vi "TLEparsing.vi"(1 "String 2":string, 2 "String":string) -> (0 "parametres_TLE":cdb[][](array[numeric]))   [LabVIEW 2015]
uses:
  <vilib>/imath/engines/lvmath/Plug In/_Char/NIMS_CH_character datatype.ctl
  <vilib>/imath/engines/lvmath2/RunTimeEngine/Managers/WorkSpace/UID Generator.vi
  <vilib>/imath/engines/lvmath/Plug In/_Char/NIMS_CH_String to Character Array.vi
  <vilib>/imath/engines/lvmath2/RunTimeEngine/RangeToken/NIMS_Range_R2 - Integer.vi
  <instcachedir>/0/NIMS_Range_R2 - Integer_396D5D4FB869421F9245109A0975AD54.lvgen/NIMS_Range_R2 - Integer_396D5D4FB869421F9245109A0975AD54_000.vi
  <vilib>/imath/engines/lvmath2/RunTimeEngine/CommandStatement/MC_CommandStatement_break.vi
  <vilib>/imath/engines/lvmath2/RunTimeEngine/IndexRead/NIMS V(S).vi
  <instcachedir>/0/NIMS V(S)_0488751826AF41519A22953C041130DC.lvgen/NIMS V(S)_0488751826AF41519A22953C041130DC_003.vi
  <vilib>/imathl/engines/lvmath/Functions/Error Handling/Create Error.vi
  <vilib>/imath/engines/lvmath2/RunTimeEngine/IndexReplace/NIMS V(S)=S.vi
  <instcachedir>/0/NIMS V(S)=S_9916D32195284AEB9D40BA9A64F3B0C5.lvgen/NIMS V(S)=S_9916D32195284AEB9D40BA9A64F3B0C5_004.vi
  <vilib>/imath/engines/lvmath2/RunTimeEngine/ErrorHandling/NIMS_Create Error From Enums.vi
  <vilib>/imath/engines/lvmath2/RunTimeEngine/BuiltInFunctions/length/NIMS_length(GV).vi
  <instcachedir>/0/NIMS_length(GV)_08A3D13377FD4E4B96F5795FBF3698FA.lvgen/NIMS_length(GV)_08A3D13377FD4E4B96F5795FBF3698FA_003.vi
  <vilib>/imath/engines/lvmath2/RunTimeEngine/IndexRead/NIMS V(R2).vi
  <instcachedir>/0/NIMS V(R2)_C76619605A0E4E9F8B2FA9389712AC47.lvgen/NIMS V(R2)_C76619605A0E4E9F8B2FA9389712AC47_002.vi
  <vilib>/imath/engines/lvmath/Plug In/_Char/NIMS_CH_Character 2D to String 1D.vi
  <vilib>/imath/engines/lvmath2/RunTimeEngine/BuiltInFunctions/str_to_num/NIMS_str_to_num.vi
  <vilib>/imath/engines/lvmath2/RunTimeEngine/RowToken/NIMS_RowToken_M_M.vi
  <instcachedir>/0/NIMS_RowToken_M_M_4D065800700C47988D760C22D4E255DD.lvgen/NIMS_RowToken_M_M_4D065800700C47988D760C22D4E255DD_003.vi
  <vilib>/imath/engines/lvmath2/RunTimeEngine/RunTimeType/NIMS_RunTimeType_From StrictType (excl LVString).vi
  <instcachedir>/0/NIMS_RunTimeType_From StrictType (excl LVString)_EB1C38A9BC5048DA9ABDA8F781E54D21.lvgen/NIMS_RunTimeType_From StrictType (excl LVString)_EB1C38A9BC5048DA9ABDA8F781E54D21_000.vi
  <vilib>/imath/engines/lvmath2/RunTimeEngine/LocalVariableDefStatement/MC_LocalVariableDefStatement_Display.vi
  <vilib>/imath/engines/lvmath2/RunTimeEngine/Managers/SymbolTable/Clear UID.vi
  <vilib>/imath/engines/lvmath2/RunTimeEngine/NodeEndStatement/NIMS_NodeEndStatement_Output.vi
  <instcachedir>/0/NIMS_NodeEndStatement_Output_53EC0D466D134D7ABD903AC30B43404B.lvgen/NIMS_NodeEndStatement_Output_53EC0D466D134D7ABD903AC30B43404B_003.vi
  <vilib>/imath/engines/lvmath2/RunTimeEngine/ErrorHandling/NIMS_Finalize Error.vi
  <vilib>/imath/engines/lvmath2/RunTimeEngine/Managers/SymbolTable/NIMS_WorkSpace.lvlib
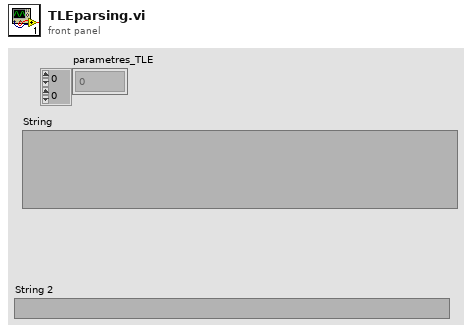
[diagram p1: front panel]
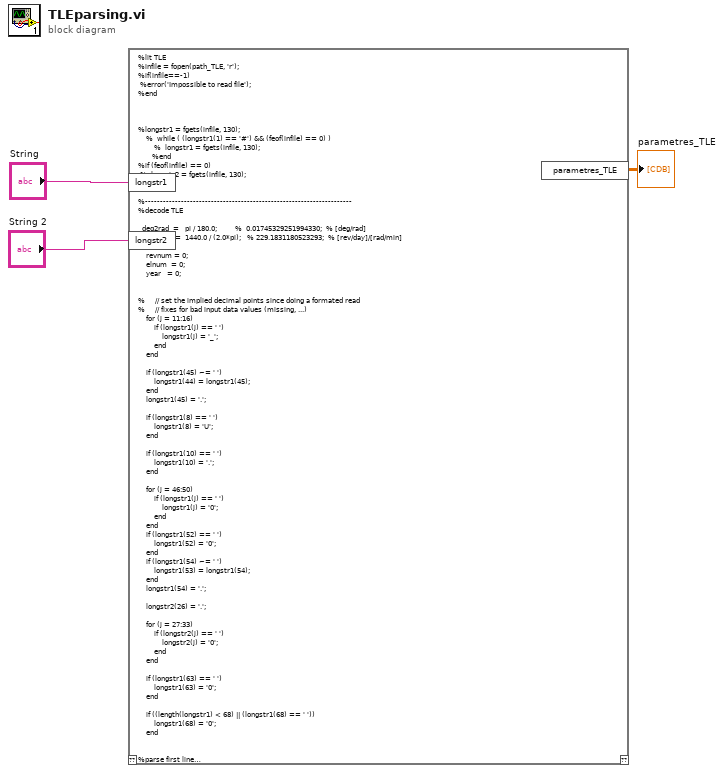
[diagram p0: block diagram]
diagram:
  n1 = mathscript code="%lit TLE\n%infile = fopen(path_TLE, 'r');\n%if(infile==-1)\n %error('Impossible to read file'); \n%end\n\n\n\n%longstr1 = fgets(infile, 130);\n    %  while ( (longstr1(1) == '#') && (feof(infile) == 0) )\n        %  longstr1 = fgets(infile, 130);\n       %end\n%if (feof(infile) == 0)            \n %  longstr2 = fgets(infile, 130);\n%end\n\n%---------------------------------------------------------------------\n%decode TLE\n\n  deg2rad  =   pi / 180.0;         %  0.01745329251994330;  % [deg/rad]\n    xpdotp   =  1440.0 / (2.0*pi);   % 229.1831180523293;  % [rev/day]/[rad/min]  \n\n    revnum = 0; \n    elnum  = 0;\n    year   = 0; \n    \n\n%     // set the implied decimal points since doing a formated read\n%     // fixes for bad input data values (missing, ...)\n    for (j = 11:16)\n        if (longstr1(j) == ' ')\n            longstr1(j) = '_';\n        end\n    end\n\n    if (longstr1(45) ~= ' ')\n        longstr1(44) = longstr1(45);\n    end\n    longstr1(45) = '.';\n     \n    if (longstr1(8) == ' ')\n        longstr1(8) = 'U';\n    end\n\n    if (longstr1(10) == ' ')\n        longstr1(10) = '.';\n    end\n\n    for (j = 46:50)\n        if (longstr1(j) == ' ')\n            longstr1(j) = '0';\n        end\n    end\n    if (longstr1(52) == ' ')\n        longstr1(52) = '0';\n    end\n    if (longstr1(54) ~= ' ')\n        longstr1(53) = longstr1(54);\n    end\n    longstr1(54) = '.';\n\n    longstr2(26) = '.';\n     \n    for (j = 27:33)\n        if (longstr2(j) == ' ')\n            longstr2(j) = '0';\n        end\n    end\n     \n    if (longstr1(63) == ' ')\n        longstr1(63) = '0';\n    end\n\n    if ((length(longstr1) < 68) || (longstr1(68) == ' '))\n        longstr1(68) = '0';\n    end\n    \n   \n%parse first line\n satnum = str2num(longstr1(3:7));\n    classification = longstr1(8);\n    intldesg = longstr1(10:17);\n  epochyr =  str2num(longstr1(19:20));\n   epochdays =  str2num(longstr1(21:32));\n    ndot = str2num(longstr1(34:43));\n    nddot =  str2num(longstr1(44:50));\n    nexp_array =  str2num(longstr1(51:52));\n    bstar =  str2num(longstr1(53:59));\n    ibexp_array =  str2num(longstr1(60:61));\n    numb_array =  str2num(longstr1(63));\n    elnum_array= str2num(longstr1(65:68));\n\n%parse second line\n\ncardnumb =  str2num(longstr2(1));\n    satnum =  str2num(longstr2(3:7));\n    inclo =  str2num(longstr2(8:16));\n    nodeo = str2num(longstr2(17:25));\n    ecco = str2num(longstr2(26:33));\n    argpo =  str2num(longstr2(34:42));\n    mo =  str2num(longstr2(43:51));\n   no = str2num(longstr2(52:63));\n    revnum_array =  str2num(longstr2(64:68));\n\n\nparametres_TLE=[satnum, epochyr, epochdays, ndot, nddot, nexp_array,bstar, ibexp_array, numb_array, elnum_array,  inclo, nodeo, ecco, argpo, mo, no, revnum_array ]\n\n%fclose(infile)" ("Nœud MathScript")("longstr1"="String", "longstr2"="String 2") -> ("parametres_TLE"=→"parametres_TLE":cdb[][])  [unwired: 1 in, 1 out]
